vi "Read XBox Controller Data.vi"(6 "Direction Info":T1, 7 "Button Info":T2, 8 "Axis Info":T3) -> (0 "B":bool, 1 "Y":bool, 2 "A":bool caption="Boolean", 3 "Steer Value Output String":string, 4 "X":bool, 5 "Drive Value Output String":string)   [LabVIEW 2011]
uses:
  _GlobalVariables&Libraries/ATV Program Global Variables.vi
panel:
  out "LB":bool
  out "Start":bool
  out "Stop/Back":bool
  out "Direction Cluster":T4
  out "RB":bool
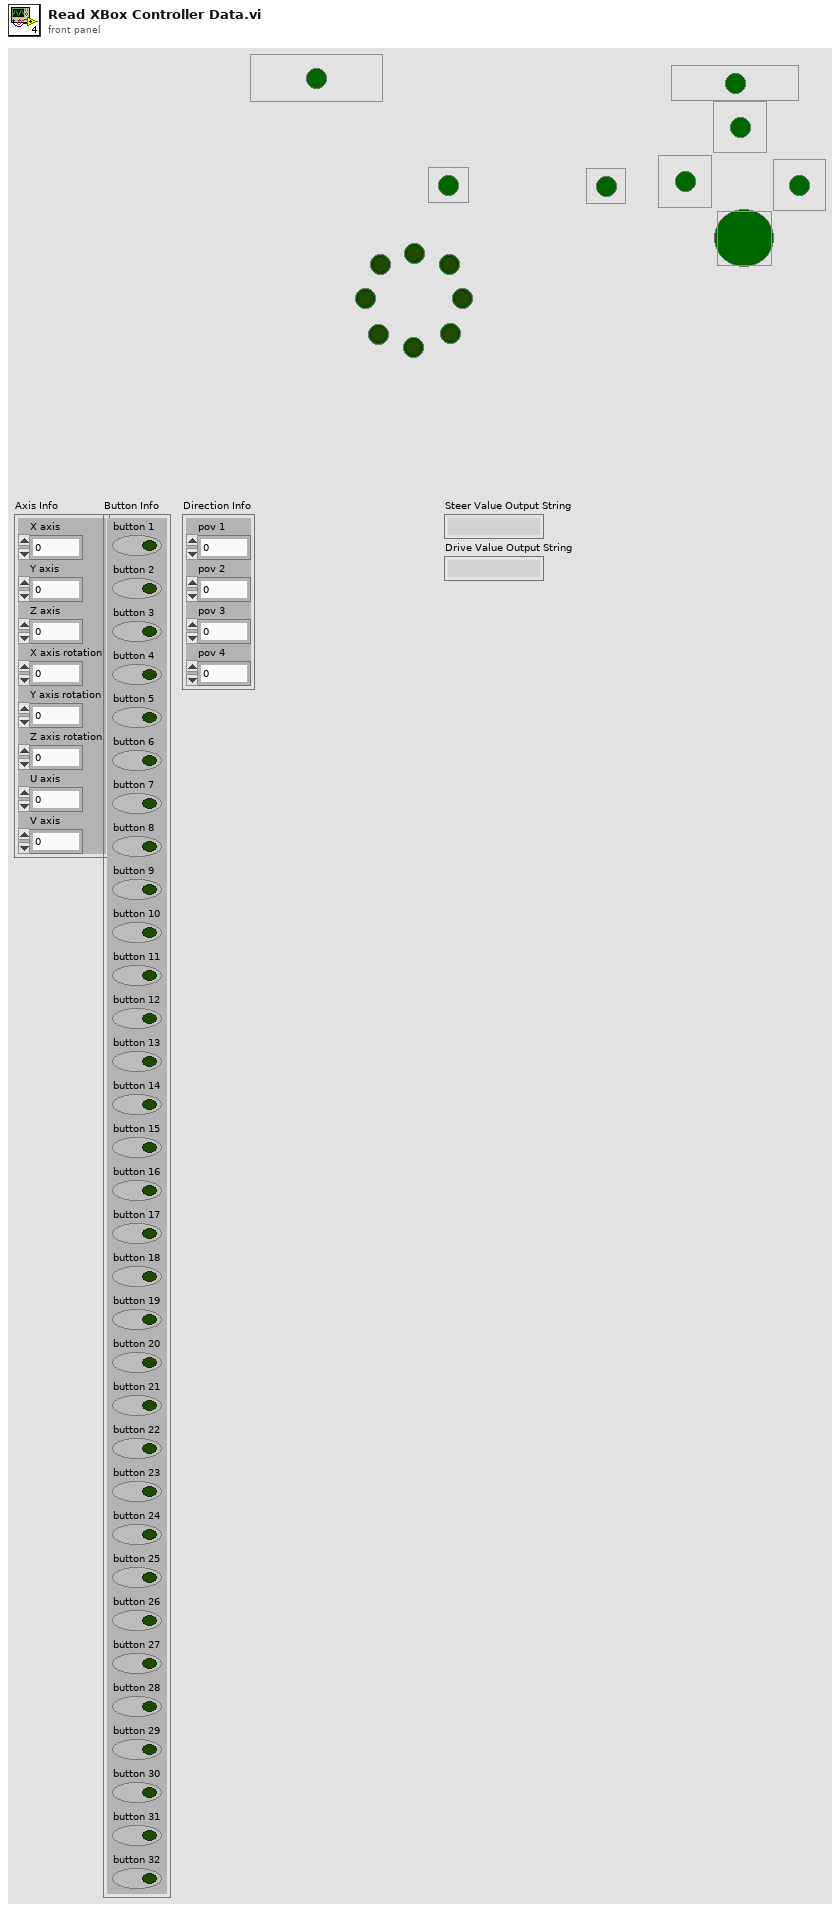
[diagram p1: front panel]
types:
  T1 = cluster{"pov 1":i32, "pov 2":i32, "pov 3":i32, "pov 4":i32}
  T2 = cluster{"button 1":bool, "button 2":bool, "button 3":bool, "button 4":bool, "button 5":bool, "button 6":bool, "button 7":bool, "button 8":bool, "button 9":bool, "button 10":bool, "button 11":bool, "button 12":bool, "button 13":bool, "button 14":bool, "button 15":bool, "button 16":bool, "button 17":bool, "button 18":bool, "button 19":bool, "button 20":bool, "button 21":bool, "button 22":bool, "button 23":bool, "button 24":bool, "button 25":bool, "button 26":bool, "button 27":bool, "button 28":bool, "button 29":bool, "button 30":bool, "button 31":bool, "button 32":bool}
  T3 = cluster{"X axis":i32, "Y axis":i32, "Z axis":i32, "X axis rotation":i32, "Y axis rotation":i32, "Z axis rotation":i32, "U axis":i32, "V axis":i32}
  T4 = cluster{"Boolean 4":bool, "Boolean 6":bool, "Boolean 3":bool, "Boolean 7":bool, "Boolean 2":bool, "Boolean 9":bool, "Boolean 5":bool, "Boolean 8":bool}
  T5 = cluster{"Drive Value Output String":string, "Steer Value Output String":string, "Button A":bool, "Button B":bool, "Error Out":errorcluster, "Disable XBox Drive & Steer":bool, "Disable XBox Controller":bool, "XBOX Button Trigger Time (ms)":u32, "Button X":bool, "Button Y":bool}
  T6 = cluster{bool, bool, bool, bool, bool, bool, bool, bool}
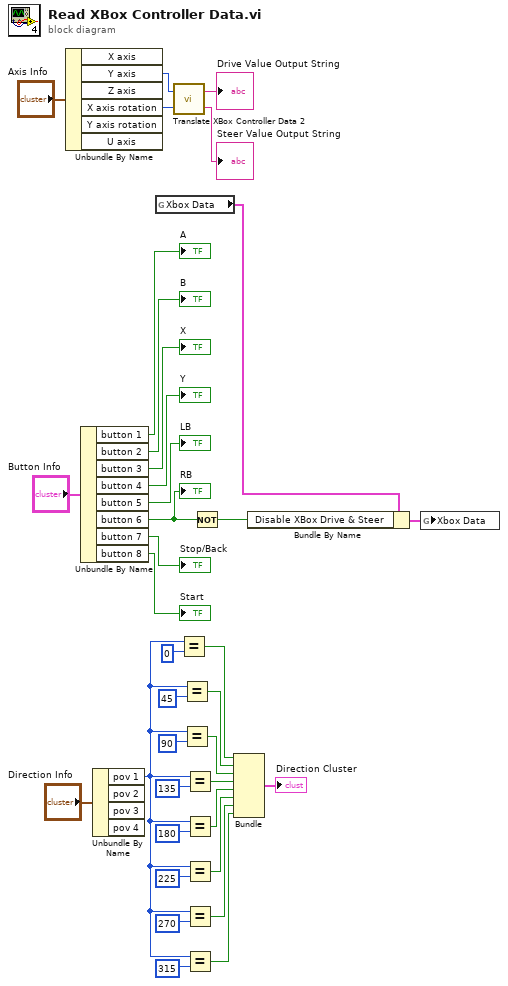
[diagram p0: block diagram]
diagram:
  n1 = Unbundle By Name("Axis Info") -> ("Y axis"=w8:i32, "X axis rotation"=w7:i32)  [unwired: 4 out]
  n2 = Unbundle By Name("Button Info") -> ("button 1"=→"A":bool, "button 2"=→"B":bool, "button 3"=→"X":bool, "button 4"=→"Y":bool, "button 5"=→"LB":bool, "button 6"=w2:bool, "button 7"=→"Stop/Back":bool, "button 8"=→"Start":bool)
  "RB" <- w2
  n3 = Unbundle By Name("Direction Info") -> ("pov 1"=w28:i32)  [unwired: 3 out]
  n4 = global read "ATV Program Global Variables.vi" "Xbox Data"() -> (w3:T5)
  n5 = call "Translate XBox Controller Data 2.vi"("Steer Axis"=w7, "Drive Axis"=w8) -> ("Steer Value Output String"=→"Steer Value Output String":string, "Drive Value Output String"=→"Drive Value Output String":string)
  n6 = Equal?(x=w28, y=0) -> (x = y?=w27:bool)
  n7 = Equal?(x=w28, y=45) -> (x = y?=w26:bool)
  n8 = Equal?(x=w28, y=90) -> (x = y?=w25:bool)
  n9 = Equal?(x=w28, y=135) -> (x = y?=w24:bool)
  n10 = Equal?(x=w28, y=180) -> (x = y?=w23:bool)
  n11 = Equal?(x=w28, y=225) -> (x = y?=w22:bool)
  n12 = Equal?(x=w28, y=270) -> (x = y?=w21:bool)
  n13 = Equal?(x=w28, y=315) -> (x = y?=w20:bool)
  n14 = Not(x=w2) -> (.not. x?=w1:bool)
  n15 = Bundle(w27, w26, w25, w24, w23, w22, w21, w20) -> (→"Direction Cluster":T6)  [unwired: 1 in]
  n16 = Bundle By Name(cluster=w3, "Disable XBox Drive & Steer"=w1) -> (w4:T5)
  n17 = global write "ATV Program Global Variables.vi" "Xbox Data"(w4) -> ()
